vi "_Update Experiment.vi"(4 "Expt#":i32, 5 "error in":errorcluster, 6 "Offset":u16, 7 "Expt":T1 {"Mass Range"."Resolution Type" items=["High/High", "Medium/Medium", "Low/Low", "High/Medium", "High/Low", "Medium/High", "Medium/Low", "Low/High", "Low/Medium"]}) -> (0 "error out":errorcluster, 1 "Next Offset":u16)   [LabVIEW 2015]
uses:
  Type/_RT Expt.ctl
  Type/_Run Mode.ctl
  Type/_RT Active Ch.ctl
  Type/_RT Mass Range.ctl
  Type/_RT Res Type.ctl
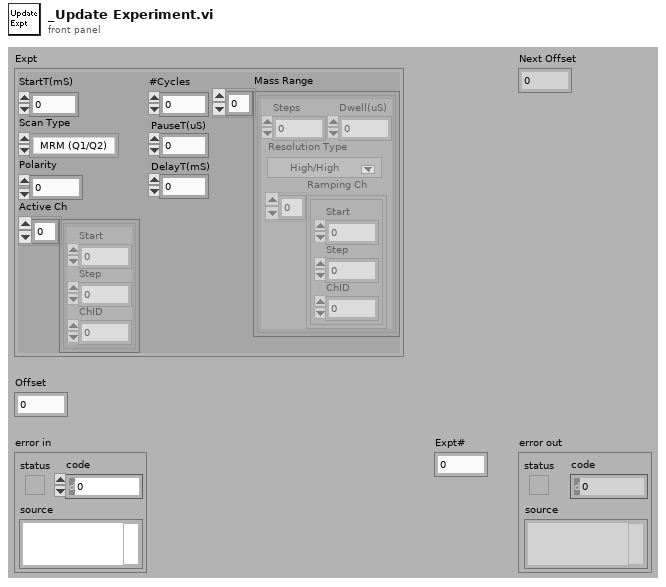
[diagram p1: front panel]
types:
  T1 = typedef "_RT Expt.ctl" = cluster{"StartT(mS)":i32, "#Cycles":i32, "Scan Type":T2, "PauseT(uS)":i32, "Polarity":u8, "DelayT(mS)":i32, "Active Ch":T3[], "Mass Range":T4[]}
  T2 = typedef "_Run Mode.ctl" = enum16{"MRM (Q1/Q2)", "Q1 Scan", "Q1 SRM", "Q2 Scan", "Q2 SRM", "Product Scan", "Precursor Scan", "Neutral Loss", "Neutral Gain"}
  T3 = typedef "_RT Active Ch.ctl" = cluster{"Start":i32, "Step":i32, "ChID":i32}
  T4 = typedef "_RT Mass Range.ctl" = cluster{"Steps":i32, "Dwell(uS)":i32, "Resolution Type":T5, "Ramping Ch":T3[]}
  T5 = typedef "_RT Res Type.ctl" = u16
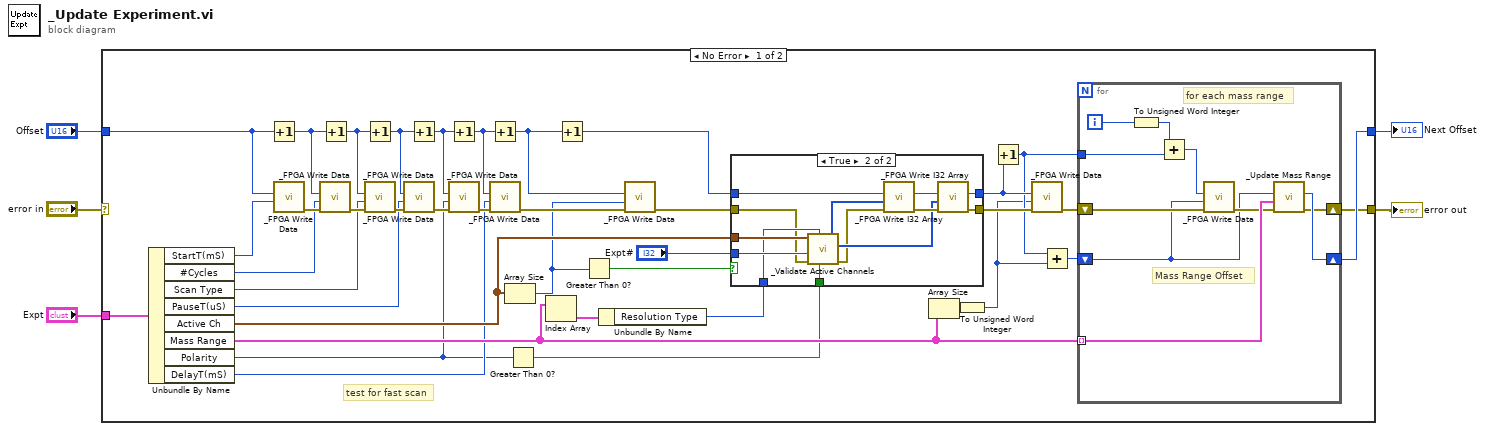
[diagram p0: block diagram]
diagram:
  n1 = case shown="No Error" "error in" {
    selector: "error in" -> [_ w71]
    tunnel: [w31 w71] -> w4
    tunnel: "Offset" -> [w33 w70]
    tunnel: [w32 w70] -> w2
    tunnel: "Expt" -> [w8 _]
    frame No Error {
      # "test for fast scan"
      n2 = Unbundle By Name(w8) -> ("StartT(mS)"=w44:i32, "#Cycles"=w42:i32, "Scan Type"=w19:T2, "PauseT(uS)"=w11:i32, "Active Ch"=w28:T3[], "Mass Range"=w22:T4[], "Polarity"=w9:u8, "DelayT(mS)"=w10:i32)
      n3 = Increment(x=w33) -> (x+1=w41:u16)
      n4 = call "_FPGA Write Data.vi"("Data"=w44, "Address"=w33) -> ("error out"=w43:errorcluster)  [unwired: 4 in, 2 out]
      n5 = call "_FPGA Write Data.vi"("error in"=w43, "Data"=w42, "Address"=w41) -> ("error out"=w25:errorcluster)  [unwired: 3 in, 2 out]
      n6 = Increment(x=w41) -> (x+1=w24:u16)
      n7 = Increment(x=w24) -> (x+1=w16:u16)
      n8 = call "_FPGA Write Data.vi"("error in"=w25, "Data"=w19, "Address"=w24) -> ("error out"=w13:errorcluster)  [unwired: 3 in, 2 out]
      n9 = call "_FPGA Write Data.vi"("error in"=w13, "Data"=w11, "Address"=w16) -> ("error out"=w17:errorcluster)  [unwired: 3 in, 2 out]
      n10 = Increment(x=w16) -> (x+1=w15:u16)
      n11 = Increment(x=w15) -> (x+1=w14:u16)
      n12 = call "_FPGA Write Data.vi"("error in"=w17, "Data"=w9, "Address"=w15) -> ("error out"=w12:errorcluster)  [unwired: 3 in, 2 out]
      n13 = Increment(x=w14) -> (x+1=w26:u16)
      n14 = call "_FPGA Write Data.vi"("error in"=w12, "Data"=w10, "Address"=w14) -> ("error out"=w27:errorcluster)  [unwired: 3 in, 2 out]
      n15 = Array Size(array=w28) -> (size(s)=w23:i32)
      n16 = Greater Than 0?(x=w9) -> (x > 0?=w18:bool)
      n17 = Index Array(array=w22) -> (element=w21:T4)  [unwired: 1 in]
      n18 = Increment(x=w26) -> (x+1=w40:u16)
      n19 = Greater Than 0?(x=w23) -> (x > 0?=w37:bool)
      n20 = Unbundle By Name(w21) -> ("Resolution Type"=w20:T5)
      n21 = call "_FPGA Write Data.vi"("error in"=w27, "Data"=w23, "Address"=w26) -> ("error out"=w39:errorcluster)  [unwired: 3 in, 2 out]
      n22 = case shown="True" w37 {
        tunnel: w40 -> [w55 w69]
        tunnel: w39 -> [w56 w59]
        tunnel: [w56 w66] -> w38
        tunnel: [w55 w65] -> w34
        tunnel: w28 -> [_ w64]
        tunnel: "Expt#" -> [_ w61]
        tunnel: w20 -> [_ w60]
        tunnel: w18 -> [_ w57]
        frame False {
        }
        frame True {
          n23 = call "_Validate Active Channels.vi"("Negative (F)"=w57, "Resolution Type"=w60, "error in"=w59, "Expt#"=w61, "Active Ch"=w64) -> ("error out"=w58:errorcluster, "DAC Values"=w62:i32[], "Ch ID"=w63:i32[])  [unwired: 1 in, 1 out]
          n24 = call "_FPGA Write I32 Array.vi"("error in"=w58, "U32 Array"=w63, "Offset (0)"=w69) -> ("error out"=w68:errorcluster, "Next Offset"=w67:u16)  [unwired: 2 in, 1 out]
          n25 = call "_FPGA Write I32 Array.vi"("error in"=w68, "U32 Array"=w62, "Offset (0)"=w67) -> ("error out"=w66:errorcluster, "Next Offset"=w65:u16)  [unwired: 2 in, 1 out]
        }
      }
      n26 = Array Size(array=w22) -> (size(s)=w7:i32)
      n27 = To Unsigned Word Integer(number=w7) -> (unsigned 16bit integer=w6:u16)
      n28 = Increment(x=w34) -> (x+1=w29:u16)
      n29 = call "_FPGA Write Data.vi"("error in"=w38, "Data"=w6, "Address"=w34) -> ("error out"=w36:errorcluster)  [unwired: 3 in, 2 out]
      n30 = Add(x=w29, y=w6) -> (x+y=w35:u16)
      n31 = for {
        shift-right: [w47] -> w31
        shift-left: w36 -> [w54]
        tunnel: w29 -> [w52]
        shift-right: [w48] -> w32
        shift-left: w35 -> [w49]
        tunnel: w22 -> [w51] mode=indexing
        i -> [w46]
        # "for each mass range"
        # "Mass Range Offset"
        n32 = To Unsigned Word Integer(number=w46) -> (unsigned 16bit integer=w45:u16)
        n33 = Add(x=w45, y=w52) -> (x+y=w53:u16)
        n34 = call "_FPGA Write Data.vi"("error in"=w54, "Data"=w49, "Address"=w53) -> ("error out"=w50:errorcluster)  [unwired: 3 in, 2 out]
        n35 = call "_Update Mass Range.vi"("error in"=w50, "Mass Range"=w51, "Offset"=w49) -> ("error out"=w47:errorcluster, "Next Offset"=w48:u16)  [unwired: 1 in, 2 out]
      }
    }
    frame Error {
    }
  }
  "error out" <- w4
  "Next Offset" <- w2
